vi "Gyro Compensated Offset.vi"(6 "Boolean":bool, 9 "Right Setpoint":dbl, 10 "Left Setpoint":dbl) -> (1 "RightCompensatedSP":dbl, 2 "LeftCompensatedSP":dbl)   [LabVIEW 2018]
uses:
  2af4d726-9e88-4db4-b186-decd53a48a63.vi
  Framework/Robot Global Data.vi
  <vilib>/addons/control/pid/pid.llb/PID (DBL).vi
  <vilib>/addons/control/pid/NI_PID_pid.lvlib
panel:
  in  "PID gains":T1={"proportional gain (Kc)"=0.01, "integral time (Ti, min)"=0.0, "derivative time (Td, min)"=0.0} {"derivative time (Td, min)" format="%.3f"; "integral time (Ti, min)" format="%.3f"; "proportional gain (Kc)" format="%.3f"}
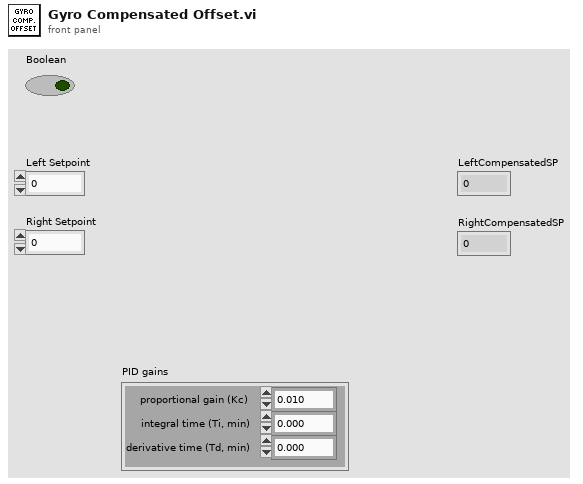
[diagram p1: front panel]
types:
  T1 = cluster{"proportional gain (Kc)":dbl, "integral time (Ti, min)":dbl, "derivative time (Td, min)":dbl}
  T2 = cluster{"X Angle":dbl, "Y Angle":dbl, "Z Angle":dbl}
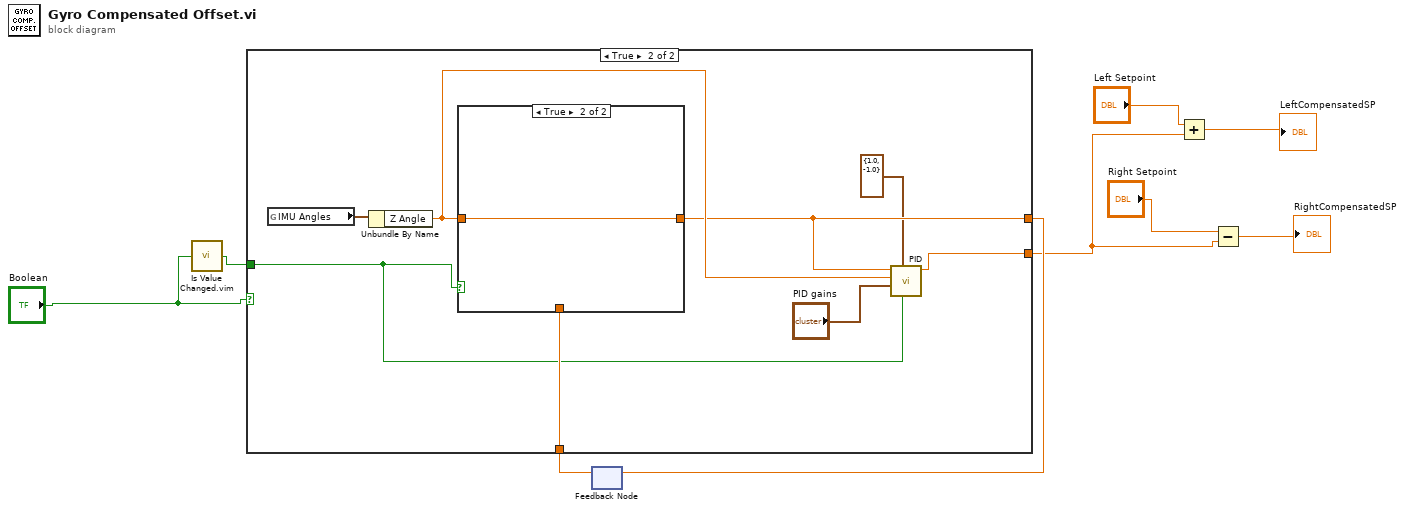
[diagram p0: block diagram]
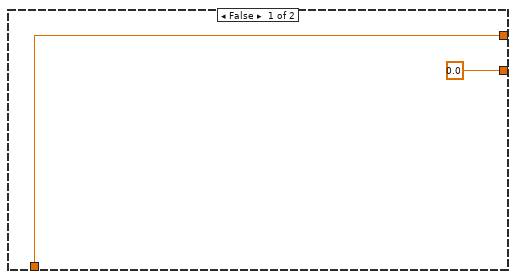
[diagram p2: hidden frame]
diagram:
  n1 = call "Is Value Changed.vim"("value"="Boolean") -> ("changed or first call?"=w1:bool)
  n2 = feedback #1() -> (w8:dbl)  [unwired: 1 in]
  n3 = case shown="True" "Boolean" {
    tunnel: [w10 w15] -> w9
    tunnel: w8 -> [w10 w18]
    tunnel: [0.0 ("output") w13] -> w3
    tunnel: w1 -> [_ w12]
    frame False {
    }
    frame True {
      n4 = global read "Robot Global Data.vi" "IMU Angles"() -> (w19:T2)
      n5 = Unbundle By Name(w19) -> ("Z Angle"=w16:dbl)
      n6 = case shown="True" w12 {
        tunnel: w16 -> [_ w21]
        tunnel: [w20 w21] -> w15
        tunnel: w18 -> [w20 _]
        frame False {
        }
        frame True {
        }
      }
      n7 = call-poly <vilib>:"PID.vi"("reinitialize? (F)"=w12, "output range"=cluster{"output high":dbl, "output low":dbl} {"output high"=1.0, "output low"=-1.0}, "PID gains"="PID gains", "process variable"=w16, "setpoint"=w15) -> ("output"=w13:dbl)  [unwired: 5 in, 1 out]
    }
  }
  n8 = feedback-in #1(w9) -> ()
  n9 = Add(x="Left Setpoint", y=w3) -> (x+y=→"LeftCompensatedSP":dbl)
  n10 = Subtract(x="Right Setpoint", y=w3) -> (x-y=→"RightCompensatedSP":dbl)
